vi "Autotest.vi"(8 "error in (no error)":errorcluster caption="entrée d'erreur (pas d'erreur)", 11 "Class Spectrum_Analyser RS306B en entrée":refnum<class "Class Spectrum_Analyser RS306B.lvclass">) -> (0 "error out":errorcluster caption="sortie d'erreur", 2 "Autotest Ok ?":bool, 3 "Class Spectrum_Analyser RS306B en sortie":refnum<class "Class Spectrum_Analyser RS306B.lvclass">)   [LabVIEW 2020, in "Library Instrument & Equipement.lvlib" / "Library Spectrum Analyser.lvlib" / "Class Spectrum_Analyser RS306B.lvclass"]
uses:
  Class Spectrum_Analyser RS306B.lvclass
  C:/Users/ngarcin/OneDrive - Altyor/Standard TB/Class/Spectrum Analyser/Class Spectrum Analyser (Default)/Class Spectrum Analyser (Default).lvclass
  Class Spectrum_Analyser RS306B.lvclass/Class Spectrum_Analyser RS306B.ctl
  user32.dll
  Library Spectrum Analyser.lvlib
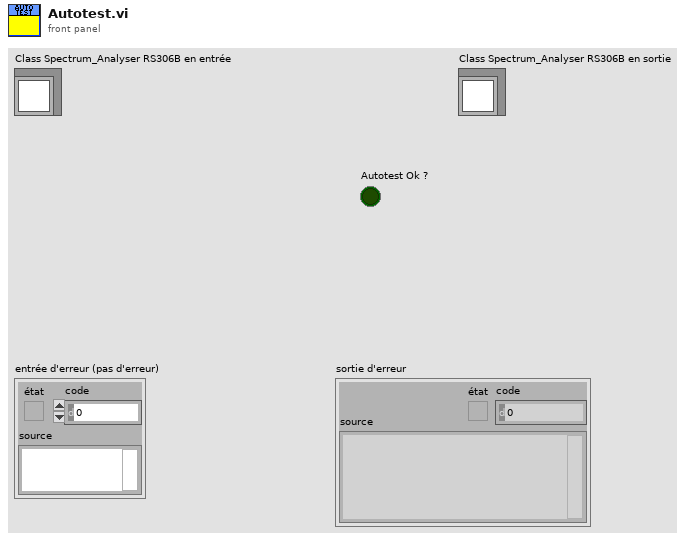
[diagram p1: front panel]
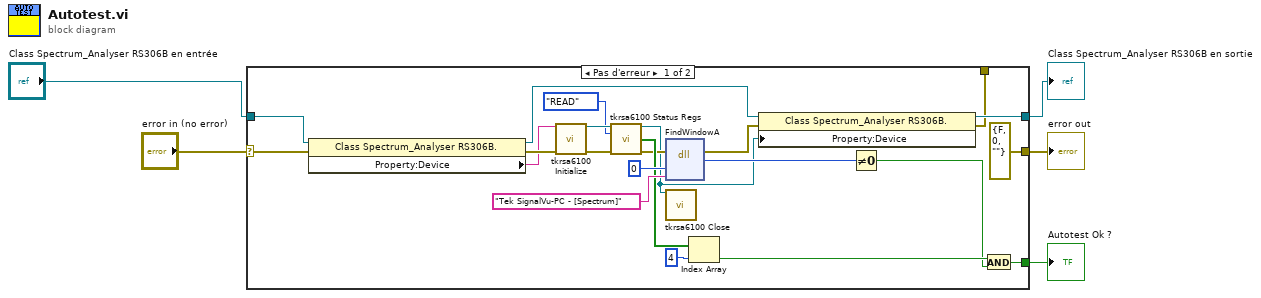
[diagram p0: block diagram]
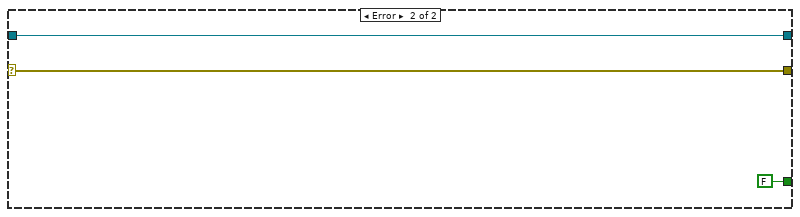
[diagram p2: hidden frame]
diagram:
  n1 = case shown="Pas d'erreur" "error in (no error)" {
    selector: "error in (no error)" -> [w15 w30]
    tunnel: [errorcluster {"status"=FALSE, "code"=0, "source"=""} ("error IO") w30] -> w4
    tunnel: [w17 FALSE] -> w3
    tunnel: [w10 w28] -> w2
    tunnel: "Class Spectrum_Analyser RS306B en entrée" -> [w13 w28]
    tunnel: [w6 _] -> _
    frame No Error {
      n2 = property class="Class Spectrum_Analyser RS306B."(reference=w13, error in=w15) -> (reference out=w12:refnum<class "Class Spectrum_Analyser RS306B.lvclass">, error out=w14:errorcluster, "Property:Device"=w8:string)
      n3 = call "tkrsa6100 Initialize.vi"("VISA Resource Name"=w8, "error in (no error)"=w14) -> ("dup VISA Resource Name"=w24:refnum<visa-resource-name>, "error out"=w23:errorcluster)  [unwired: 9 in, 3 out]
      n4 = call "tkrsa6100 Status Regs.vi"("VISA Resource Name"=w24, "Set/Read\nStatus Register (SET)"=enum16{"SET", "READ"}."READ" ("Set/Read\nStatus Register (SET)"), "error in (no error)"=w23) -> ("dup VISA Resource Name"=w9:refnum<visa-resource-name>, "Register Bits Array"=w22:bool[], "error out"=w16:errorcluster)  [unwired: 8 in, 2 out]
      n5 = dll-call lib="user32.dll" fn="FindWindowA" label="FindWindow"(error in=w16, "lpszClassName"=0, "lpszWindowName"="Tek SignalVu-PC - [Spectrum]") -> (error out=w11:errorcluster, "hWnd"=w25:u32)  [unwired: 4 in, 1 out]
      n6 = call "tkrsa6100 Close.vi"("VISA Resource Name"=w9) -> ()  [unwired: 14 in, 1 out]
      n7 = Index Array(array=w22, index=4 ("indice")) -> (element=w19:bool)
      n8 = property class="Class Spectrum_Analyser RS306B."(reference=w12, error in=w11, "Property:Device"=w9) -> (reference out=w10:refnum<class "Class Spectrum_Analyser RS306B.lvclass">, error out=w6:errorcluster)
      n9 = Not Equal To 0?(x=w25) -> (x != 0?=w18:bool)
      n10 = And(x=w19, y=w18) -> (x .and. y?=w17:bool)
    }
    frame Error {
    }
  }
  "error out" <- w4
  "Class Spectrum_Analyser RS306B en sortie" <- w2
  "Autotest Ok ?" <- w3
